vi "GetControlLabel.vi"(6 "error in":errorcluster, 9 "Control in":refnum<class "Control.lvclass">) -> (0 "error out":errorcluster, 3 "Control out":refnum<class "Control.lvclass">, 4 "Items":T1[](array[typedef]))   [LabVIEW 2014, in "PythonConverter_GUI.lvclass"]
uses:
  PythonConverter_GUI.lvclass
  VI Interpreter/Classes/Control/Control.lvclass
  PythonConfiguration/TypeDefs/ItemTD.ctl
  VI Interpreter/Classes/Control/Control.lvclass/Control.ctl
  VI Interpreter/Classes/Decoration/Decoration.lvclass/Decoration.ctl
  VI Interpreter/Classes/Text/Text.lvclass/Text.ctl
  VI Interpreter/Classes/GObject/GObject.lvclass/GObject.ctl
  VI Interpreter/Classes/Text/Text.lvclass
  VI Interpreter/Classes/GObject/GObject.lvclass
  PythonConfiguration/PythonConfiguration.lvclass
  VI Interpreter/Classes/Decoration/Decoration.lvclass
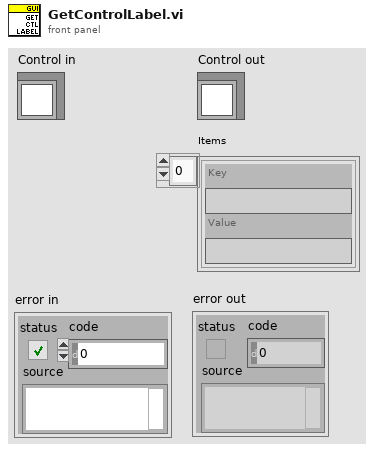
[diagram p1: front panel]
types:
  T1 = typedef "PythonConfiguration.lvclass/ItemTD.ctl" = cluster{"Key":string, "Value":string}
  T2 = typedef "LVFontTypeDef.ctl" = cluster{"Font Name":string, "Size":u16, "Bold":bool, "Italic":bool, "Underline":bool, "Strikeout":bool, "Color":u32}
  T3 = typedef "LVRectTypeDef.ctl" = cluster{"Left":i16, "Top":i16, "Right":i16, "Bottom":i16}
  T4 = typedef "LVPositionTypeDef.ctl" = cluster{"Left":i32, "Top":i32}
  T5 = typedef "LVBoundsTypeDef.ctl" = cluster{"Width":u32, "Height":u32}
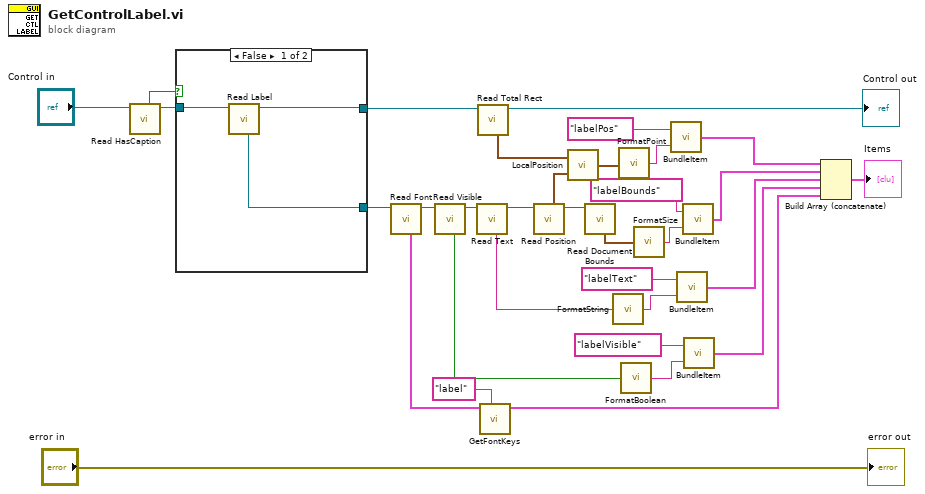
[diagram p0: block diagram]
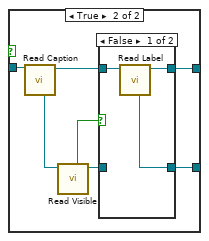
[diagram p2: hidden frame]
diagram:
  n1 = call "Read HasCaption.vi"("Control in"="Control in") -> ("Control out"=w31:refnum<class "Control.lvclass">, "HasCaption"=w32:bool)  [unwired: 7 in]
  n2 = case shown="False" w32 {
    tunnel: w31 -> [w36 w43]
    tunnel: [w34 w39] -> w11
    tunnel: [w35 w40] -> w30
    frame False {
      n3 = call "Read Label.vi"("Control in"=w36) -> ("Control out"=w35:refnum<class "Control.lvclass">, "Label"=w34:refnum<class "Text.lvclass">)  [unwired: 7 in]
    }
    frame True {
      n4 = call "Read Caption.vi"("Control in"=w43) -> ("Control out"=w41:refnum<class "Control.lvclass">, "Caption"=w42:refnum<class "Text.lvclass">)  [unwired: 7 in]
      n5 = call "Read Visible.vi"("Decoration in"=w42) -> ("Decoration out"=w38:refnum<class "Text.lvclass">, "Visible"=w37:bool)  [unwired: 7 in]
      n6 = case shown="False" w37 {
        tunnel: w41 -> [w46 w48]
        tunnel: [w45 w48] -> w40
        tunnel: [w44 w47] -> w39
        tunnel: w38 -> [_ w47]
        frame False {
          n7 = call "Read Label.vi"("Control in"=w46) -> ("Control out"=w45:refnum<class "Control.lvclass">, "Label"=w44:refnum<class "Text.lvclass">)  [unwired: 7 in]
        }
        frame True {
        }
      }
    }
  }
  n8 = call "Read Font.vi"("Text in"=w11) -> ("Text out"=w10:refnum<class "Text.lvclass">, "Font"=w9:T2)  [unwired: 7 in]
  n9 = call "Read Visible.vi"("Decoration in"=w10) -> ("Decoration out"=w16:refnum<class "Text.lvclass">, "Visible"=w12:bool)  [unwired: 7 in]
  n10 = call "Read Text.vi"("Text in"=w16) -> ("Text out"=w29:refnum<class "Text.lvclass">, "Text"=w24:string)  [unwired: 7 in]
  n11 = call "Read Total Rect.vi"("GObject in"=w30) -> ("GObject out"=→"Control out":refnum<class "Control.lvclass">, "Total Rect"=w19:T3)  [unwired: 7 in]
  n12 = call "GetFontKeys.vi"("name"="label", "Font"=w9) -> ("font items"=w7:T1[])  [unwired: 7 in]
  n13 = call "Read Position.vi"("GObject in"=w29) -> ("GObject out"=w6:refnum<class "Text.lvclass">, "Position"=w18:T4)  [unwired: 7 in]
  n14 = call "LocalPosition.vi"("Position"=w18, "Total Bounds Rect"=w19) -> ("Local Position"=w17:T4)
  n15 = call "Read Document Bounds.vi"("Text in"=w6) -> ("Document Bounds"=w5:T5)  [unwired: 7 in, 1 out]
  n16 = call "FormatString.vi"("String"=w24) -> ("value"=w23:string)  [unwired: 1 in]
  n17 = call "FormatPoint.vi"("point"=w17) -> ("value"=w26:string)
  n18 = call "FormatBoolean.vi"("boolean"=w12) -> ("value"=w13:string)
  n19 = call "FormatSize.vi"("size"=w5) -> ("value"=w3:string)
  n20 = call "BundleItem.vi"("Value"=w26, "Key"="labelPos") -> ("Item"=w4:T1)
  n21 = call "BundleItem.vi"("Value"=w23, "Key"="labelText") -> ("Item"=w21:T1)
  n22 = call "BundleItem.vi"("Value"=w3, "Key"="labelBounds") -> ("Item"=w2:T1)
  n23 = call "BundleItem.vi"("Value"=w13, "Key"="labelVisible") -> ("Item"=w14:T1)
  n24 = Build Array (concatenate)(w4, w2, w21, w14, w7) -> (→"Items":T1[])
  "error out" <- "error in"
